vi "move_to_ir.vi"(0 "step":i32, 1 "precision":dbl, 2 "target_ir_r":dbl, 3 "samples":i32, 4 "delay_after":u32, 5 "target_ir_l":dbl) -> ()   [LabVIEW 2017]
uses:
  <vilib>/myRIO/Instrument Drivers/Onboard IO/AI/typedefs/AI Reference.ctl
  <vilib>/myRIO/Common/Instrument Driver Framework/Utilities/typedefs/myRIO Generic Hardware Reference.ctl
  <vilib>/myRIO/Common/Instrument Driver Framework/Utilities/typedefs/Hardware Version Enum.ctl
  <vilib>/myRIO/Common/Instrument Driver Framework/Utilities/typedefs/myRIO v1.0 Reference.ctl
  <vilib>/myRIO/Common/Instrument Driver Framework/Utilities/typedefs/Generic FPGA Reference.ctl
  <vilib>/myRIO/Common/Instrument Driver Framework/myRIO v1.0/AI/typedefs/AI Channels List.ctl
  <vilib>/myRIO/Common/Instrument Driver Framework/myRIO v1.0/AI/typedefs/AI Channels Enum.ctl
  <vilib>/myRIO/Common/Instrument Driver Framework/Utilities/typedefs/Analog Scaling Constants List.ctl
  <vilib>/myRIO/Common/Instrument Driver Framework/Utilities/typedefs/Analog Scaling Constants.ctl
  <vilib>/userdefined/High Color/nirio_resource_hc.ctl
  <vilib>/myRIO/Common/Instrument Driver Framework/Utilities/vis/Is FPGA Ref Available.vi
  <vilib>/myRIO/Common/Instrument Driver Framework/myRIO v1.0/AI/vis/myRIO v1.1 Open AI.vi
  <vilib>/myRIO/Instrument Drivers/Onboard IO/AI/vis/Read.vi
  <vilib>/Analysis/baseanly.llb/Mean (DBL).vi
  <vilib>/myRIO/Common/Instrument Driver Framework/Utilities/vis/Validate Channels.vi
  <vilib>/myRIO/Common/Instrument Driver Framework/myRIO v1.0/AI/vis/myRIO v1.0 Reserve AI.vi
  <vilib>/myRIO/Common/Instrument Driver Framework/myRIO v1.0/AI/vis/myRIO v1.0 Build MUX Configuration AI.vi
  <vilib>/myRIO/Common/Instrument Driver Framework/myRIO v1.0/Resource Manager/vis/myRIO v1.0 Reserve Channel List.vi
  <vilib>/myRIO/Common/Instrument Driver Framework/myRIO v1.0/Resource Manager/vis/myRIO v1.0 Reserve Channel.vi
  <vilib>/myRIO/Common/Instrument Driver Framework/myRIO v1.0/Resource Manager/vis/myRIO v1.0 Unreserve Channel.vi
  <vilib>/myRIO/Common/Instrument Driver Framework/myRIO v1.0/Resource Manager/vis/myRIO v1.0 Build Mutex Name.vi
  <vilib>/Utility/VariantDataType/GetNumericInfo.vi
  <vilib>/Utility/error.llb/Error Cluster From Error Code.vi
  <vilib>/myRIO/Common/Instrument Driver Framework/myRIO v1.0/myRIO v1.1 Open.vi
  <vilib>/myRIO/Common/Instrument Driver Framework/myRIO v1.0/AI/vis/myRIO v1.0 Get Scaling Constants AI.vi
  <vilib>/myRIO/Common/Instrument Driver Framework/Utilities/vis/IO Manager.vi
  <vilib>/myRIO/Common/Instrument Driver Framework/Utilities/vis/Configuration Manager.vi
  <vilib>/myRIO/Common/Instrument Driver Framework/myRIO v1.0/myRIO v1.0 Close.vi
  <vilib>/myRIO/Common/Instrument Driver Framework/myRIO v1.0/AI/vis/myRIO v1.0 Read AI.vi
  GlobalVar.vi
  <vilib>/myRIO/Express VI/Onboard IO/AI/AI Express VI.xnode
  <vilib>/myRIO/Instrument Drivers/Onboard IO/AI/vis/myRIO AI Open.xnode
  <vilib>/Analysis/NI_AALBase.lvlib
  <vilib>/myRIO/Instrument Drivers/Onboard IO/AI/AI.lvlib
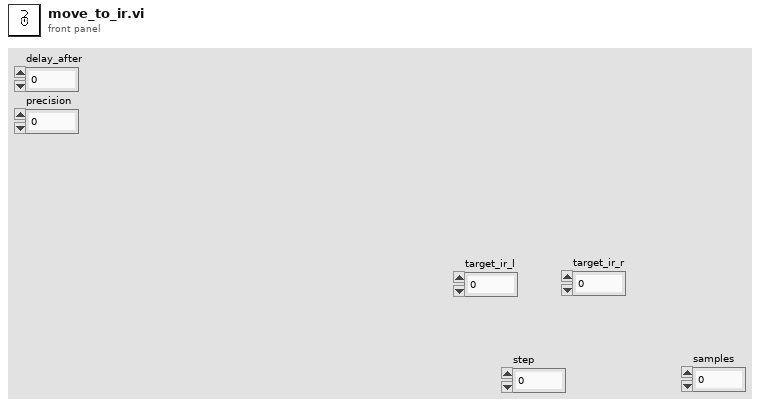
[diagram p1: front panel]
types:
  T1 = typedef "AI.lvlib/AI Reference.ctl" = cluster{"myRIO Reference":T2, "AI Channels List":T6, "AI Scaling Constants List":T8}
  T2 = typedef "myRIO Generic Hardware Reference.ctl" = cluster{"myRIO Model":T3, "myRIO Hardware Reference":T4}
  T3 = typedef "Hardware Version Enum.ctl" = enum16{"Unknown", "myRIO-1900", "myRIO-1950", "roboRIO", "NI ELVIS RIO CM"}
  T4 = typedef "myRIO v1.0 Reference.ctl" = cluster{"Generic FPGA Reference":T5, "Allow multiple opens":bool}
  T5 = typedef "Generic FPGA Reference.ctl" = refnum<k20>
  T6 = typedef "AI Channels List.ctl" = T7[]
  T7 = typedef "AI Channels Enum.ctl" = enum16{"Not Connected", "AudioIn/Left", "AudioIn/Right", "C/AI0", "C/AI1", "A/AI0", "A/AI1", "A/AI2", "A/AI3", "B/AI0", "B/AI1", "B/AI2", "B/AI3", "AI/AI0", "AI/AI1", "AI/AI2", "AI/AI3"}
  T8 = typedef "Analog Scaling Constants List.ctl" = T9[]
  T9 = typedef "Analog Scaling Constants.ctl" = cluster{"LSB Weight (Volts)":dbl, "Offset (Volts)":dbl, "Signed?":bool}
  T10 = typedef "nirio_resource_hc.ctl" = tag
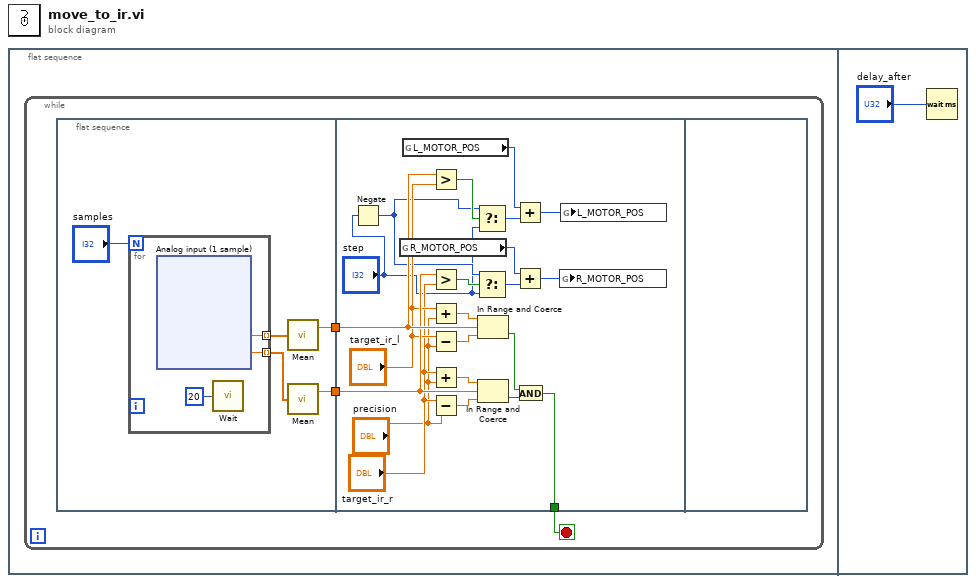
[diagram p0: block diagram]
diagram:
  n1 = flat-sequence {
    frame #0 {
      n2 = while {
        stop <- w1 stop-if-true
        n3 = flat-sequence {
          tunnel: [w6] -> w3
          tunnel: [w5] -> w2
          tunnel: w3 -> [w63]
          tunnel: w2 -> [w62]
          tunnel: [w53] -> w1
          frame #0 {
            n4 = for {
              N: "samples" -> [_]
              tunnel: [w11] -> w7 mode=indexing
              tunnel: [w10] -> w4 mode=indexing
              n5 = xnode "Analog input (1 sample)"() -> ("l (B/AI0 (Pin 3))"=w11:dbl, "r (B/AI1 (Pin 5))"=w10:dbl)  [unwired: 1 in, 1 out]
              n6 = call "Wait"("Count(uSec)"=u32 20) -> ()  [unwired: 1 out]
            }
            n7 = call-poly <vilib>:"Mean.vi"("X"=w7) -> ("mean"=w6:dbl)  [unwired: 1 out]
            n8 = call-poly <vilib>:"Mean.vi"("X"=w4) -> ("mean"=w5:dbl)  [unwired: 1 out]
          }
          frame #1 {
            n9 = Negate(x="step") -> (-x=w51:i32)
            n10 = global read "GlobalVar.vi" "R_MOTOR_POS"() -> (w67:i32)
            n11 = global read "GlobalVar.vi" "L_MOTOR_POS"() -> (w69:i32)
            n12 = Greater?(x=w63, y="target_ir_l") -> (0:w65:bool)
            n13 = Greater?(x=w62, y="target_ir_r") -> (0:w64:bool)
            n14 = Add(x="target_ir_l", y="precision") -> (x+y=w60:dbl)
            n15 = Subtract(x="target_ir_l", y="precision") -> (x-y=w61:dbl)
            n16 = Add(x="target_ir_r", y="precision") -> (x+y=w59:dbl)
            n17 = Subtract(x="target_ir_r", y="precision") -> (x-y=w58:dbl)
            n18 = Select(t=w51, s=w65, f="step") -> (s? t:f=w70:i32)
            n19 = Select(t=w51, s=w64, f="step") -> (s? t:f=w68:i32)
            n20 = In Range and Coerce(upper limit=w60, x=w63, lower limit=w61) -> (In Range?=w55:bool)  [unwired: 1 out]
            n21 = In Range and Coerce(upper limit=w59, x=w62, lower limit=w58) -> (In Range?=w54:bool)  [unwired: 1 out]
            n22 = Add(x=w69, y=w70) -> (x+y=w71:i32)
            n23 = Add(x=w67, y=w68) -> (x+y=w66:i32)
            n24 = And(x=w55, y=w54) -> (x .and. y?=w53:bool)
            n25 = global write "GlobalVar.vi" "R_MOTOR_POS"(w66) -> ()
            n26 = global write "GlobalVar.vi" "L_MOTOR_POS"(w71) -> ()
          }
          frame #2 {
          }
        }
      }
    }
    frame #1 {
      n27 = Wait (ms)(milliseconds to wait="delay_after") -> ()  [unwired: 1 out]
    }
  }
